vi "Achizitie continua.vi"(5 "Numãrul de repetari":dbl=-1.0, 6 "Bluetooth":refnum<visa-resource-name>="COM3", 7 "error in (no error)":errorcluster, 8 "Perioada achizitie [s]":dbl=2.0 format="%#_13g", 9 "Numarul persoanei":ext, 10 "Alegere Modul":u16(ring) items=["Stationare", "Mers normal", "Alergare", "Cadere", "Mers labartat"]) -> (0 "error out":errorcluster, 3 "Timer":dbl)   [LabVIEW 2018]
uses:
  <vilib>/Instr/_visa.llb/VISA Configure Serial Port (Instr).vi
  <vilib>/Utility/file.llb/Write Delimited Spreadsheet (string).vi
  <vilib>/Utility/file.llb/Write Delimited Spreadsheet (I64).vi
panel:
  in  "Clear Screen":bool
  out "Calibration":T1
  out "read buffer":string
  out "transposed array":i16[][](array[numeric])
  in  "Frecventa de esantionare [Hz]":dbl=50.0
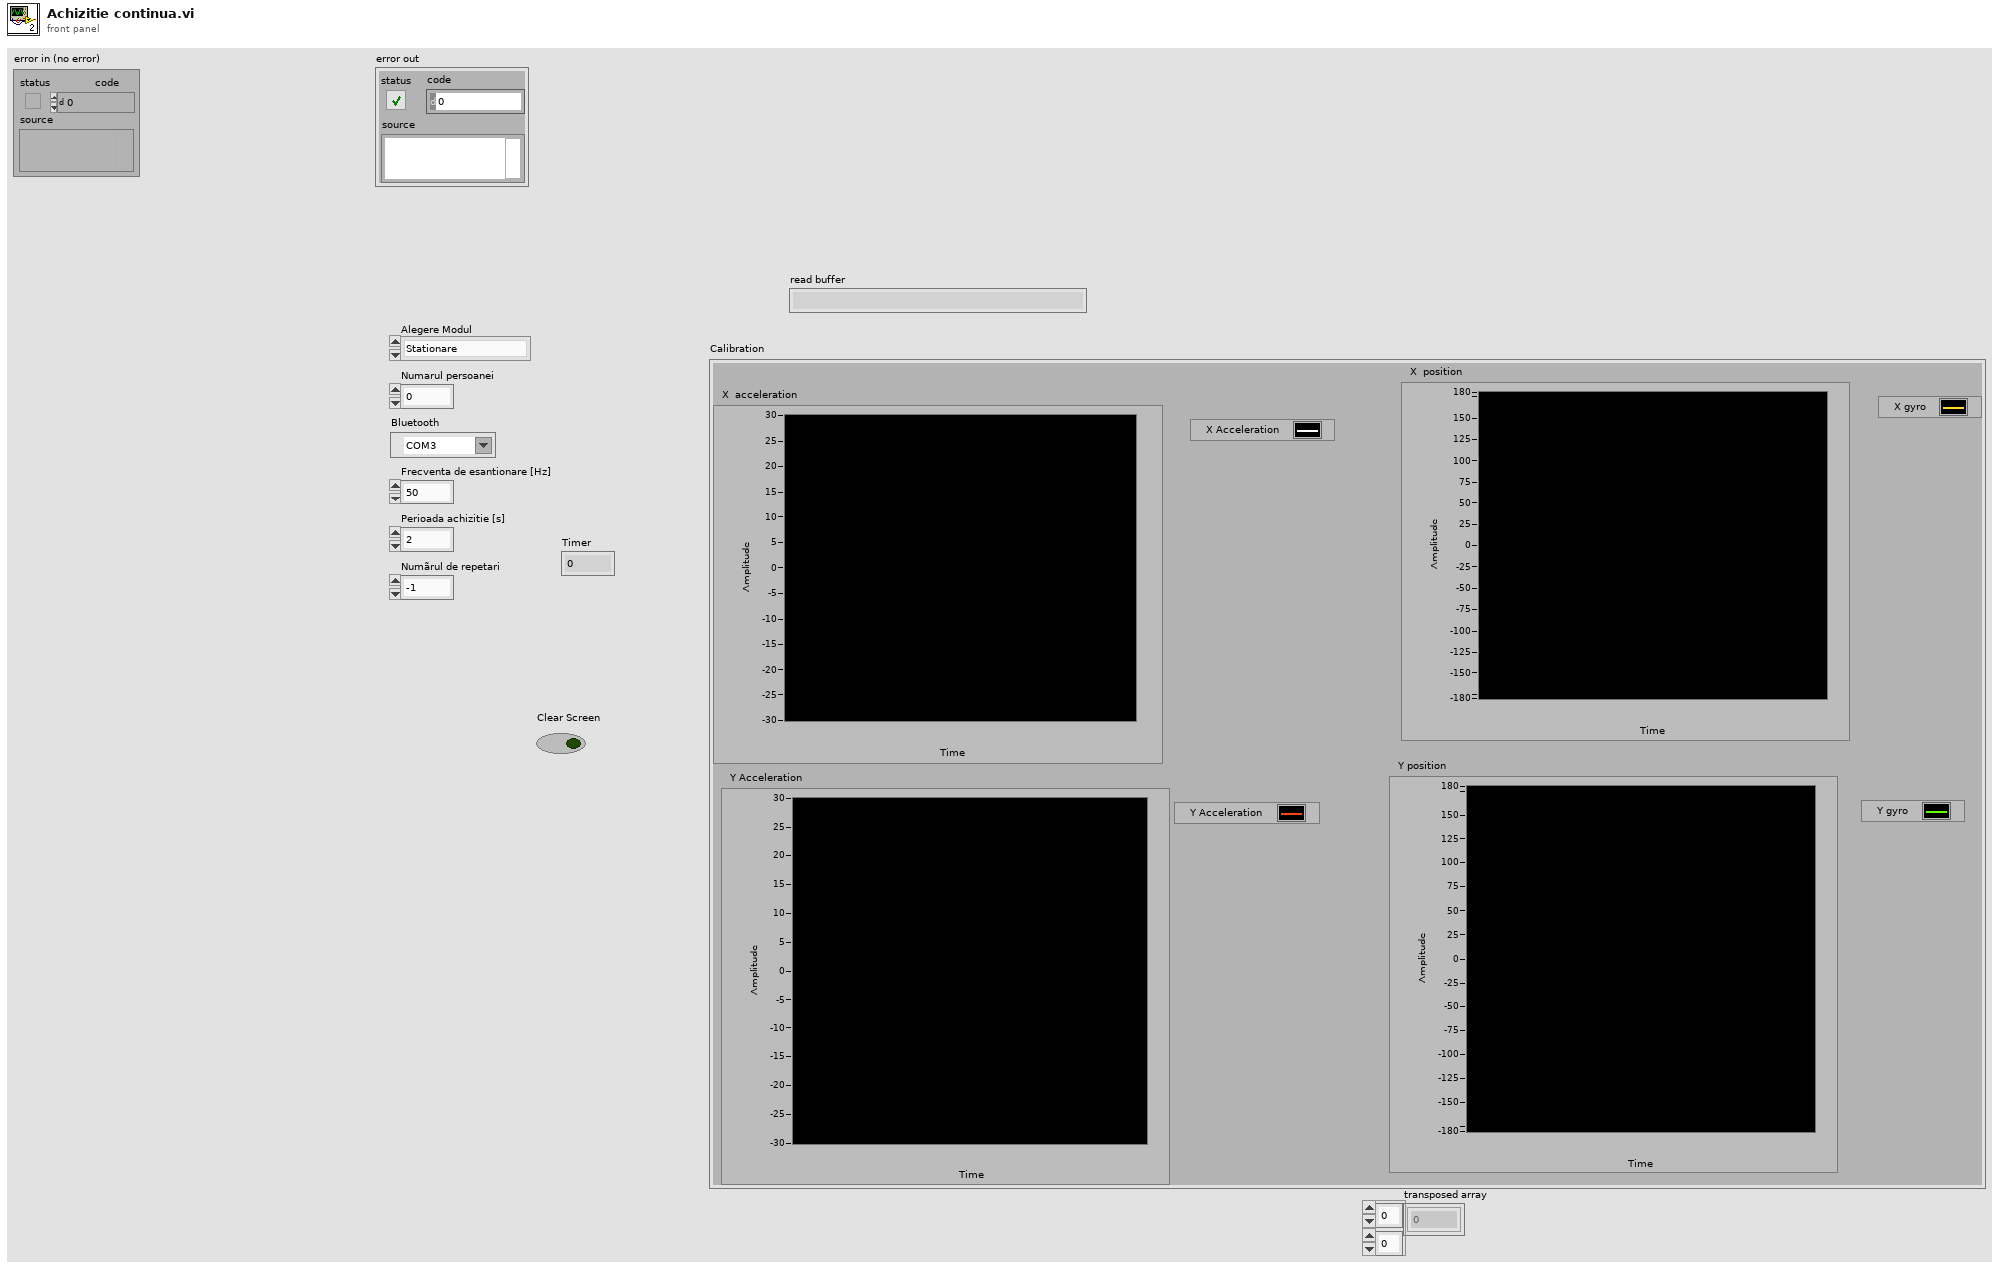
[diagram p1: front panel]
types:
  T1 = cluster{"X  acceleration":dbl, "Y Acceleration":dbl, "X  position":dbl, "Y position":dbl}
  T2 = typedef "imagedata.ctl" = cluster{"image type":i32, "image depth":i32, "image":u8[], "mask":u8[], "colors":u32[], "Rectangle":cluster{"left":i16, "top":i16, "right":i16, "bottom":i16}}
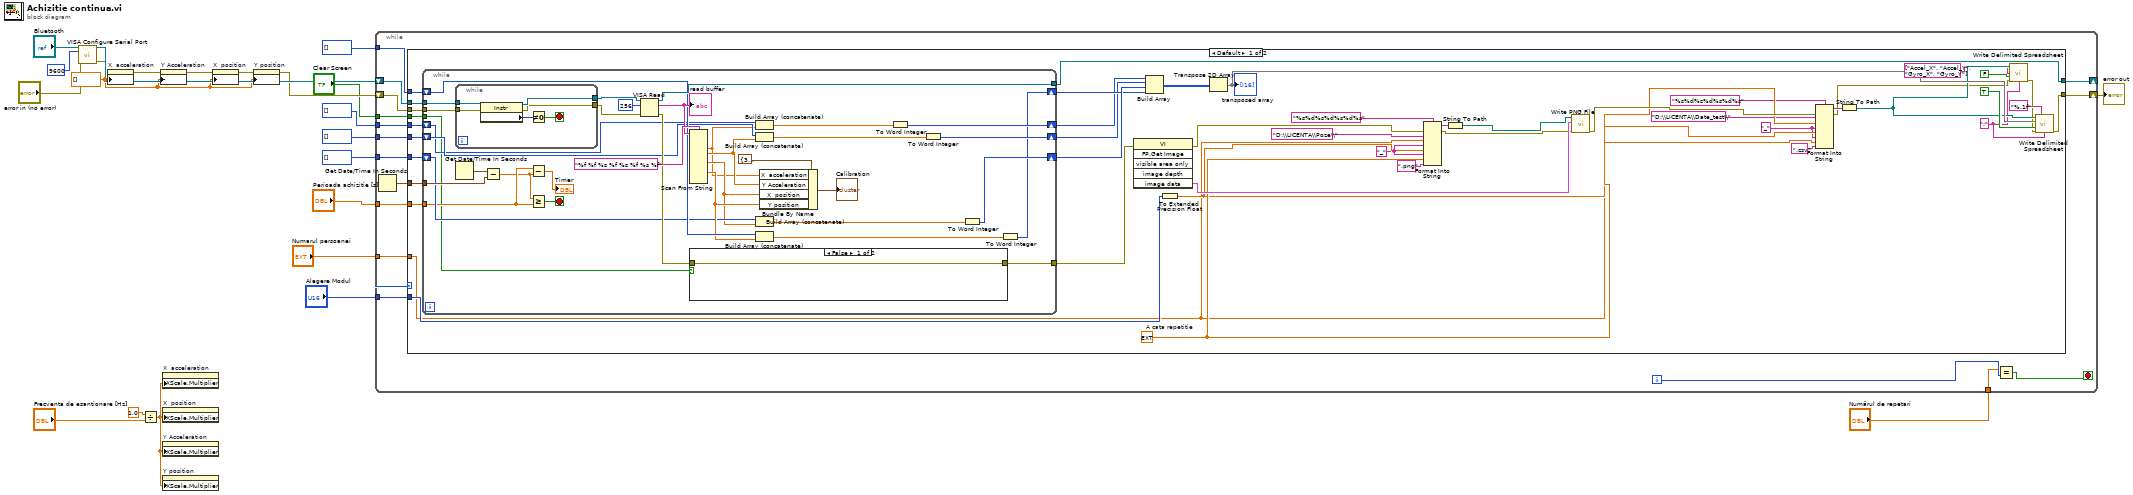
[diagram p0: block diagram]
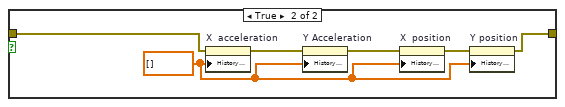
[diagram p2: hidden frame]
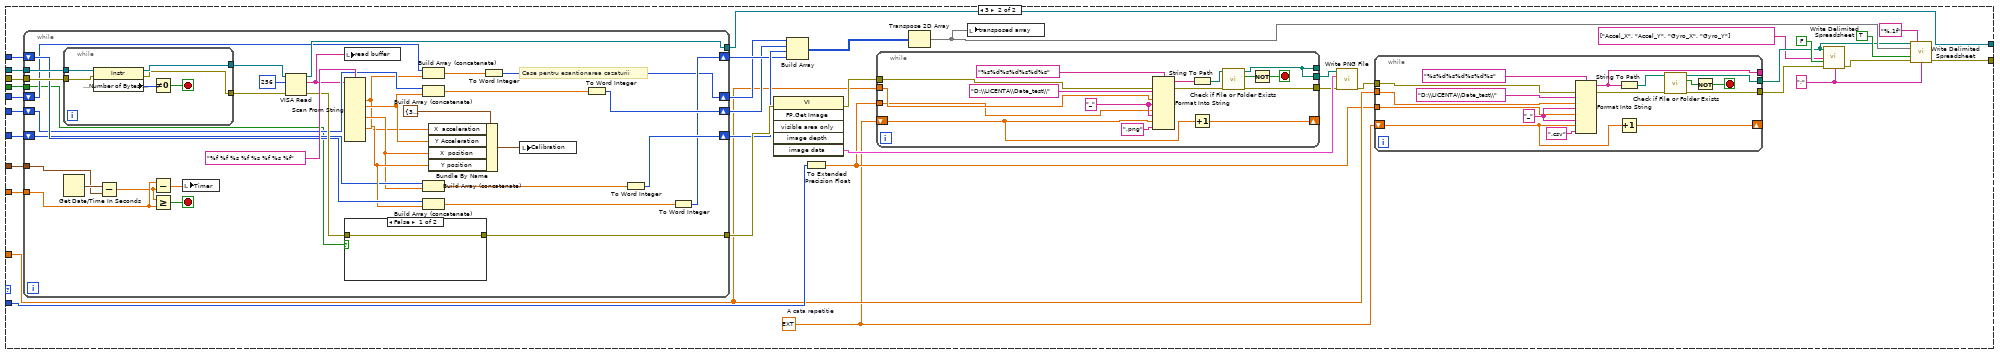
[diagram p3: hidden frame]
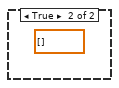
[diagram p4: hidden frame]
diagram:
  w15 = dbl[] [] ("History Data")
  n1 = call-poly "VISA Configure Serial Port"("VISA resource name"="Bluetooth", "baud rate (9600)"=u32 9600, "error in (no error)"="error in (no error)") -> ("VISA resource name out"=w21:refnum<visa-resource-name>, "error out"=w20:errorcluster)  [unwired: 11 in]
  n2 = property on="X  acceleration" class="WFChart (strict)"(error in=w20, "History Data"=w15) -> (error out=w19:errorcluster)  [unwired: 1 in, 1 out]
  n3 = Divide(x=1.0, y="Frecventa de esantionare [Hz]") -> (x/y=w14:dbl)
  n4 = property on="Y Acceleration" class="WFChart (strict)"(error in=w19, "History Data"=w15) -> (error out=w18:errorcluster)  [unwired: 1 in, 1 out]
  n5 = property on="X  acceleration" class="WFChart (strict)"("XScale.Multiplier"=w14) -> ()  [unwired: 2 in, 2 out]
  n6 = property on="X  position" class="WFChart (strict)"("XScale.Multiplier"=w14) -> ()  [unwired: 2 in, 2 out]
  n7 = property on="Y Acceleration" class="WFChart (strict)"("XScale.Multiplier"=w14) -> ()  [unwired: 2 in, 2 out]
  n8 = property on="Y position" class="WFChart (strict)"("XScale.Multiplier"=w14) -> ()  [unwired: 2 in, 2 out]
  n9 = property on="X  position" class="WFChart (strict)"(error in=w18, "History Data"=w15) -> (error out=w17:errorcluster)  [unwired: 1 in, 1 out]
  n10 = property on="Y position" class="WFChart (strict)"(error in=w17, "History Data"=w15) -> (error out=w16:errorcluster)  [unwired: 1 in, 1 out]
  n11 = while {
    tunnel: i16[] [] -> [w37]
    tunnel: i16[] [] -> [w36]
    tunnel: i16[] [] -> [w35]
    tunnel: i16[] [] -> [w34]
    tunnel: "Alegere Modul" -> [w31]
    tunnel: "Clear Screen" -> [w30]
    tunnel: "Numarul persoanei" -> [w29]
    tunnel: "Perioada achizitie [s]" -> [w28]
    shift-right: [w32] -> _
    shift-left: w21 -> [w39]
    shift-right: [w33] -> w1
    shift-left: w16 -> [w38]
    tunnel: "Numãrul de repetari" -> [w24]
    i -> [w25]
    stop <- w26 stop-if-true
    n12 = Get Date/Time In Seconds() -> (seconds since 1Jan1904=w27:timestamp)
    n13 = case shown="Default" w31 {
      tunnel: w39 -> [w84 w167]
      tunnel: w38 -> [w83 w166]
      tunnel: w27 -> [w80 w163]
      tunnel: w28 -> [w79 w162]
      tunnel: w31 -> [w73 w157]
      tunnel: w37 -> [w66 w151]
      tunnel: w36 -> [w65 w150]
      tunnel: w35 -> [w64 w149]
      tunnel: w34 -> [w63 w148]
      tunnel: [w56 w133] -> w33
      tunnel: [w55 w143] -> w32
      tunnel: w30 -> [w54 w142]
      tunnel: w29 -> [w53 w137]
      frame Default {
        w44 = "_"
        w49 = "_"
        w67 = ext 0.0  # A cata repetitie
        w61 = ";" ("delimiter (\\t)")
        n14 = while {
          tunnel: w83 -> [w114]
          tunnel: w84 -> [w113]
          tunnel: [w109] -> w82
          tunnel: [w117] -> w55
          shift-right: [w86] -> w77
          shift-left: w63 -> [w108]
          tunnel: w80 -> [w104]
          tunnel: w79 -> [w94]
          shift-right: [w88] -> w78
          shift-left: w64 -> [w102]
          shift-right: [w89] -> w57
          shift-left: w65 -> [w98]
          shift-right: [w90] -> w58
          shift-left: w66 -> [w99]
          tunnel: w54 -> [w85]
          stop <- w103 stop-if-true
          n15 = while {
            tunnel: w114 -> [w132]
            tunnel: w113 -> [w131]
            tunnel: [w130] -> w112
            tunnel: [w129] -> w111
            stop <- w128 stop-if-true
            n16 = property class="Instr"(reference=w131, error in=w132) -> (reference out=w130:refnum<visa-resource-name>, error out=w129:errorcluster, "Serial Settings:Number of Bytes at Serial Port"=w127:u32)
            n17 = Not Equal To 0?(x=w127) -> (x != 0?=w128:bool)
          }
          n18 = Get Date/Time In Seconds() -> (seconds since 1Jan1904=w105:timestamp)
          n19 = Subtract(x=w105, y=w104) -> (x-y=w93:dbl)
          n20 = Subtract(x=w94, y=w93) -> (x-y=→"Timer":dbl)
          n21 = Greater Or Equal?(x=w93, y=w94) -> (x >= y?=w103:bool)
          n22 = VISA Read(VISA resource name=w112, byte count=u32 256, error in (no error)=w111) -> (VISA resource name out=w117:refnum<visa-resource-name>, read buffer=w115:string, error out=w110:errorcluster)  [unwired: 1 out]
          "read buffer" <- w115
          n23 = Scan From String(format string="%f %f %s %f %s %f %s %f", input string=w115) -> (output 1=w96:dbl, output 2=w97:dbl, output 4=w100:dbl, output 6=w107:dbl)  [unwired: 14 in, 3 out]
          n24 = case shown="False" w85 {
            tunnel: w110 -> [w120 w122]
            tunnel: [w120 w121] -> w109
            frame False {
            }
            frame True {
              w126 = dbl[] [] ("History Data")
              n25 = property on="X  acceleration" class="WFChart (strict)"(error in=w122, "History Data"=w126) -> (error out=w123:errorcluster)  [unwired: 1 in, 1 out]
              n26 = property on="Y Acceleration" class="WFChart (strict)"(error in=w123, "History Data"=w126) -> (error out=w124:errorcluster)  [unwired: 1 in, 1 out]
              n27 = property on="X  position" class="WFChart (strict)"(error in=w124, "History Data"=w126) -> (error out=w125:errorcluster)  [unwired: 1 in, 1 out]
              n28 = property on="Y position" class="WFChart (strict)"(error in=w125, "History Data"=w126) -> (error out=w121:errorcluster)  [unwired: 1 in, 1 out]
            }
          }
          n29 = Build Array (concatenate)(w98, w96) -> (w95:dbl[])
          n30 = Build Array (concatenate)(w99, w97) -> (w91:dbl[])
          n31 = Build Array (concatenate)(w102, w100) -> (w101:dbl[])
          n32 = Build Array (concatenate)(w108, w107) -> (w87:dbl[])
          n33 = Bundle By Name(cluster=T1 {"X  acceleration"=39.0, "Y Acceleration"=-79.0, "X  position"=180.0, "Y position"=92.0} ("Calibration"), "X  acceleration"=w96, "Y Acceleration"=w97, "X  position"=w100, "Y position"=w107) -> (→"Calibration":T1)
          n34 = To Word Integer(number=w95) -> (16bit integer=w89:i16[])
          n35 = To Word Integer(number=w91) -> (16bit integer=w90:i16[])
          n36 = To Word Integer(number=w101) -> (16bit integer=w88:i16[])
          n37 = To Word Integer(number=w87) -> (16bit integer=w86:i16[])
        }
        n38 = invoke class="VI" method="FP.Get Image"(error in=w82) -> (error out=w70:errorcluster, "image data"=w81:T2)  [unwired: 5 in, 4 out]
        n39 = Build Array(w57, w58, w78, w77) -> (w76:i16[][])
        n40 = To Extended Precision Float(1:w73) -> (0:w59:ext)
        n41 = Transpose 2D Array(2D array=w76) -> (transposed array=w75:i16[][])
        "transposed array" <- w75
        n42 = Format Into String(format string="%s%d%s%d%s%d%s", error in=w70, "D:\\LICENTA\\Poze\\", w53, w49, w59, w49, w67, ".png" ("input 7")) -> (resulting string=w48:string, error out=w69:errorcluster)  [unwired: 1 in]
        n43 = String To Path(string=w48) -> (path=w68:path)
        n44 = call <vilib>:"Write PNG File.vi"("error in (no error)"=w69, "image data"=w81, "path to PNG file"=w68) -> ("error out"=w71:errorcluster)  [unwired: 7 in, 1 out]
        n45 = Format Into String(format string="%s%d%s%d%s%d%s", error in=w71, "D:\\LICENTA\\Date_test\\", w53, w44, w59, w44, w67, ".csv" ("input 7")) -> (resulting string=w43:string, error out=w41:errorcluster)  [unwired: 1 in]
        n46 = String To Path(string=w43) -> (path=w62:path)
        n47 = call-poly <vilib>:"Write Delimited Spreadsheet.vi"("file path (dialog if empty)"=w62, "1D data"=string[] ["Accel_X", "Accel_Y", "Gyro_X", "Gyro_Y"] ("Array"), "append to file? (new file:F)"=FALSE, "error in (no error)"=w41, "delimiter (\\t)"=w61) -> ("error out"=w40:errorcluster)  [unwired: 9 in, 1 out]
        n48 = call-poly <vilib>:"Write Delimited Spreadsheet.vi"("file path (dialog if empty)"=w62, "format (%d)"="%.1f" ("format (%.3f)"), "2D data"=w75, "append to file? (new file:F)"=TRUE, "error in (no error)"=w40, "delimiter (\\t)"=w61) -> ("error out"=w56:errorcluster)  [unwired: 8 in, 1 out]
      }
      frame 3 {
        w135 = ext 1.0  # A cata repetitie
        w147 = ";" ("delimiter (\\t)")
        n49 = while {
          tunnel: w166 -> [w230]
          tunnel: w167 -> [w229]
          tunnel: [w225] -> w165
          tunnel: [w232] -> w143
          shift-right: [w206] -> w160
          shift-left: w148 -> [w224]
          tunnel: w163 -> [w221]
          tunnel: w162 -> [w212]
          shift-right: [w208] -> w161
          shift-left: w149 -> [w219]
          shift-right: [w202] -> w144
          shift-left: w150 -> [w215]
          shift-right: [w209] -> w145
          shift-left: w151 -> [w216]
          tunnel: w142 -> [w203]
          stop <- w220 stop-if-true
          # "Case pentru esantionarea cazaturii"
          n50 = while {
            tunnel: w230 -> [w241]
            tunnel: w229 -> [w240]
            tunnel: [w239] -> w228
            tunnel: [w238] -> w227
            stop <- w237 stop-if-true
            n51 = property class="Instr"(reference=w240, error in=w241) -> (reference out=w239:refnum<visa-resource-name>, error out=w238:errorcluster, "Serial Settings:Number of Bytes at Serial Port"=w236:u32)
            n52 = Not Equal To 0?(x=w236) -> (x != 0?=w237:bool)
          }
          n53 = Get Date/Time In Seconds() -> (seconds since 1Jan1904=w222:timestamp)
          n54 = Subtract(x=w222, y=w221) -> (x-y=w211:dbl)
          n55 = Subtract(x=w212, y=w211) -> (x-y=w204:dbl)
          n56 = Greater Or Equal?(x=w211, y=w212) -> (x >= y?=w220:bool)
          n57 = local write "Timer"(w204) -> ()
          n58 = VISA Read(VISA resource name=w228, byte count=u32 256, error in (no error)=w227) -> (VISA resource name out=w232:refnum<visa-resource-name>, read buffer=w200:string, error out=w226:errorcluster)  [unwired: 1 out]
          n59 = local write "read buffer"(w200) -> ()
          n60 = Scan From String(format string="%f %f %s %f %s %f %s %f", input string=w200) -> (output 1=w201:dbl, output 2=w214:dbl, output 4=w217:dbl, output 6=w223:dbl)  [unwired: 14 in, 3 out]
          n61 = case shown="False" w203 {
            tunnel: w226 -> [w235 _]
            tunnel: [w235 _] -> w225
            frame False {
            }
            frame True {
              (unwired) dbl[] [] ("History Data")
            }
          }
          n62 = Build Array (concatenate)(w215, w201) -> (w213:dbl[])
          n63 = Build Array (concatenate)(w216, w214) -> (w210:dbl[])
          n64 = Build Array (concatenate)(w219, w217) -> (w218:dbl[])
          n65 = Build Array (concatenate)(w224, w223) -> (w207:dbl[])
          n66 = Bundle By Name(cluster=T1 {"X  acceleration"=39.0, "Y Acceleration"=-79.0, "X  position"=180.0, "Y position"=92.0} ("Calibration"), "X  acceleration"=w201, "Y Acceleration"=w214, "X  position"=w217, "Y position"=w223) -> (w205:T1)
          n67 = To Word Integer(number=w213) -> (16bit integer=w202:i16[])
          n68 = local write "Calibration"(w205) -> ()
          n69 = To Word Integer(number=w210) -> (16bit integer=w209:i16[])
          n70 = To Word Integer(number=w218) -> (16bit integer=w208:i16[])
          n71 = To Word Integer(number=w207) -> (16bit integer=w206:i16[])
        }
        n72 = invoke class="VI" method="FP.Get Image"(error in=w165) -> (error out=w154:errorcluster, "image data"=w164:T2)  [unwired: 5 in, 4 out]
        n73 = Build Array(w144, w145, w161, w160) -> (w159:i16[][])
        n74 = To Extended Precision Float(1:w157) -> (0:w136:ext)
        n75 = while {
          tunnel: w137 -> [w182]
          tunnel: w136 -> [w179]
          shift-right: [w172] -> _
          shift-left: w135 -> [w173]
          tunnel: [w171] -> w153
          tunnel: w154 -> [w170]
          tunnel: [w168] -> _
          tunnel: [w168] -> w152
          stop <- w175 stop-if-true
          w180 = "_"
          n76 = Format Into String(format string="%s%d%s%d%s%d%s", error in=w170, "D:\\LICENTA\\Date_test\\", w182, w180, w179, w180, w173, ".png" ("input 7")) -> (resulting string=w178:string, error out=w174:errorcluster)  [unwired: 1 in]
          n77 = String To Path(string=w178) -> (path=w177:path)
          n78 = Increment(x=w173) -> (x+1=w172:ext)
          n79 = call <vilib>:"Check if File or Folder Exists.vi"("error in (no error)"=w174, "path"=w177) -> ("error out"=w171:errorcluster, "file or folder exists?"=w176:bool, "dup path"=w168:path)  [unwired: 7 in]
          n80 = Not(x=w176) -> (.not. x?=w175:bool)
        }
        n81 = Transpose 2D Array(2D array=w159) -> (transposed array=w141:i16[][])
        n82 = local write "transposed array"(w141) -> ()
        n83 = call <vilib>:"Write PNG File.vi"("error in (no error)"=w153, "image data"=w164, "path to PNG file"=w152) -> ("error out"=w155:errorcluster)  [unwired: 7 in, 1 out]
        n84 = while {
          tunnel: w137 -> [w198]
          tunnel: w136 -> [w195]
          shift-right: [w189] -> _
          shift-left: w135 -> [w190]
          tunnel: [w188] -> w138
          tunnel: w155 -> [w187]
          tunnel: [w186] -> w140
          tunnel: [w184] -> _
          stop <- w192 stop-if-true
          w196 = "_"
          n85 = Format Into String(format string="%s%d%s%d%s%d%s", error in=w187, "D:\\LICENTA\\Date_test\\", w198, w196, w195, w196, w190, ".csv" ("input 7")) -> (resulting string=w184:string, error out=w191:errorcluster)  [unwired: 1 in]
          n86 = String To Path(string=w184) -> (path=w194:path)
          n87 = Increment(x=w190) -> (x+1=w189:ext)
          n88 = call <vilib>:"Check if File or Folder Exists.vi"("error in (no error)"=w191, "path"=w194) -> ("error out"=w188:errorcluster, "file or folder exists?"=w193:bool, "dup path"=w186:path)  [unwired: 7 in]
          n89 = Not(x=w193) -> (.not. x?=w192:bool)
        }
        n90 = call-poly <vilib>:"Write Delimited Spreadsheet.vi"("file path (dialog if empty)"=w140, "1D data"=string[] ["Accel_X", "Accel_Y", "Gyro_X", "Gyro_Y"] ("Array"), "append to file? (new file:F)"=FALSE, "error in (no error)"=w138, "delimiter (\\t)"=w147) -> ("error out"=w139:errorcluster)  [unwired: 9 in, 1 out]
        n91 = call-poly <vilib>:"Write Delimited Spreadsheet.vi"("file path (dialog if empty)"=w140, "format (%d)"="%.1f" ("format (%.3f)"), "2D data"=w141, "append to file? (new file:F)"=TRUE, "error in (no error)"=w139, "delimiter (\\t)"=w147) -> ("error out"=w133:errorcluster)  [unwired: 8 in, 1 out]
      }
    }
    n92 = Equal?(x=w24, y=w25) -> (x = y?=w26:bool)
  }
  "error out" <- w1
